vi "PPG_ABC.set letter time.vi"(0 "i ref in":refnum<vi>, 1 "letter":string, 2 "time [us]":dbl, 3 "ms timeout [ms]":i32=10000, 4 "patternGroup":i32, 5 "error in (no error)":errorcluster) -> (14 "i ref out":refnum<vi>, 17 "timed out":bool, 19 "error out":errorcluster)   [LabVIEW 2014, in "PPG_ABC.lvlib"]
doc: "Recalculates and reloads actual patterns for given letter and time. This routine can only by used, after patterns have been loaded using the method \"LoadABC\"."
uses:
  PPG_ABC.lvlib
  CS_Core/CSSystem/CoreDefs/CoreDefs.error_type.ctl
  CS_Core/CSSystem/CoreDefs/CoreDefs.error_severity.ctl
  CS_Core/CSSystem/CoreLib/CoreLib.lvlib
  CSlibraries/UtilityLib/UtilityLib.lvlib
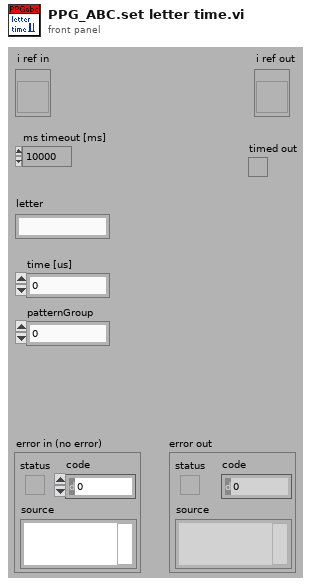
[diagram p1: front panel]
types:
  T1 = typedef "CoreDefs.error_severity.ctl" = enum16{"undefined", "information", "warning", "error", "fatal"}
  T2 = typedef "CoreDefs.error_type.ctl" = enum16{"no error", "can't load process", "can't unload process", "process does not exist", "can't install process", "can't remove process", "unknown function", "time out", "can't execute function", "duplicate queue name", "super not found", "caller queue invalid", "can't ping process", "unknown error", "VISA Error", "VISA timeout", "GPIB timeout", "GPIB error", "communication error", "data type mismatch", "can't read data from OPC server", "can't write data to OPC server", "OET error", "function not implemented", "process already exists", "invalid Shared Variable name", "error writing Shared Variable", "error reading Shared Variable", "invalid client name", "corrupt database", "unknown class", "call not authorized", "parameter out of range", "OET timeout: can't get data to modify", "invalid queue name", "requested operation incompatible with current state", "event undefined", "event disabled", "state undefined", "caller is not a friend", "EventBuilder: bad eventID", "EventBuilder: no DAQ devices", "a thread must not stop itself", "UNUSED ELEMENT4", "DiscArchiver: eventData incomplete", "DiscArchiver: eventData does not belong to run", "DiscArchiver: can't open file", "DiscArchiver: can't write to file", "DiscArchiver: available disc space low", "can't acquire semaphore", "error reading data from database", "notifier object is not existing", "can't register process", "can't unregister process", "illegal event type", "object disabled", "object already exists", "can't change state", "Instrument not found", "no connection to remote node", "invalid reference", "N/A", "UNUSED ELEMENT 1", "element not found", "illegal TCP/IP connection detected", "object does not exist", "invalid access ID", "unknown CS system", "invalid privilige", "unsupported data type", "unsupported server type", "IO server already exists", "Shared Variable already exists"}
  T3 = typedef "PPG_ABC.lvlib/PPG_ABC.i attribute.ctl" = cluster{"patternGroups":T4[], "defaultLetter":string, "defaultPatternGroup":i32, "PGRunning":T5, "PGRunningID":i32, "pgStarting":T6}
  T4 = typedef "PPG_ABC.lvlib/PPG_ABC.PG_dataType.ctl" = cluster{"PGDevice":string, "rawPatternData":cluster{"triggerCondition":i32, "timeTable":dbl[], "channelTable":string[]}[]}
  T5 = typedef "PPG_ABC.lvlib/PPG_ABC.PG_Running.ctl" = i32
  T6 = typedef "Semaphore RefNum" = refnum<k1>
  T7 = cluster{"triggerCondition":i32, "timeTable":dbl[], "channelTable":string[]}[]
  T8 = cluster{"triggerCondition":i32, "timeTable":dbl[], "channelTable":string[]}
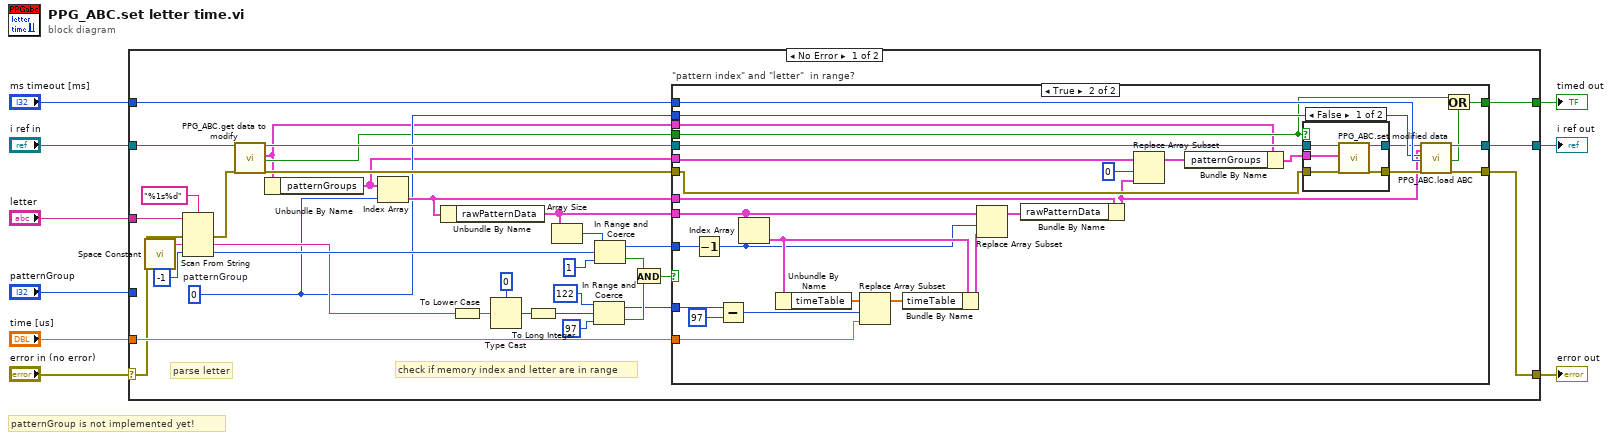
[diagram p0: block diagram]
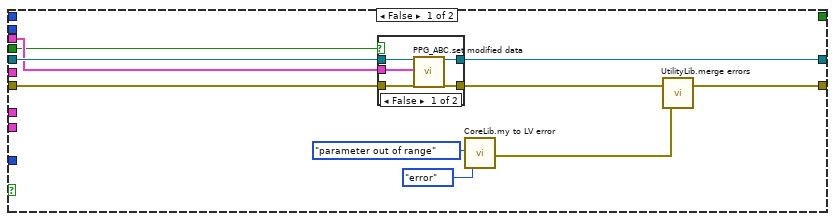
[diagram p2: hidden frame]
diagram:
  # "patternGroup is not implemented yet!"
  n1 = case shown="No Error" "error in (no error)" {
    selector: "error in (no error)" -> [w13 w100]
    tunnel: [w22 w100] -> w8
    tunnel: "i ref in" -> [w40 w99]
    tunnel: [w24 w99] -> w6
    tunnel: "ms timeout [ms]" -> [w20 _]
    tunnel: "letter" -> [w44 _]
    tunnel: "time [us]" -> [w21 _]
    tunnel: [w19 _] -> w2
    tunnel: "patternGroup" -> [_ _]
    frame No Error {
      w14 = 0  # patternGroup
      # "check if memory index and letter are in range"
      # "parse letter"
      n2 = call <vilib>:"Space Constant.vi"() -> ("String"=w42:string)
      n3 = Scan From String(format string="%1s%d", input string=w44, error in=w13, default 1=w42, default 2=-1 ("default value 2")) -> (error out=w38:errorcluster, output 1=w33:string, output 2=w35:i32)  [unwired: 1 in, 2 out]
      n4 = call "PPG_ABC.get data to modify.vi"("i ref in"=w40, "error in (no error)"=w38) -> ("i ref out"=w39:refnum<vi>, "i attribute"=w10:T3, "timed out"=w12:bool, "error out"=w23:errorcluster)  [unwired: 14 in]
      n5 = Unbundle By Name(w10) -> ("patternGroups"=w11:T4[])
      n6 = Index Array(array=w11, index=w14) -> (element=w15:T4)
      n7 = Unbundle By Name(w15) -> ("rawPatternData"=w16:T7)
      n8 = To Lower Case(string=w33) -> (all lower case string=w18:string)
      n9 = Type Cast(type=u8 0, x=w18) -> (*(type *) &x=w32:u8)
      n10 = To Long Integer(number=w32) -> (32bit integer=w17:i32)
      n11 = Array Size(array=w16) -> (size(s)=w37:i32)
      n12 = In Range and Coerce(upper limit=122, x=w17, lower limit=97) -> (coerced(x)=w25:i32, In Range?=w26:bool)
      n13 = In Range and Coerce(upper limit=w37, x=w35, lower limit=1) -> (coerced(x)=w34:i32, In Range?=w27:bool)
      n14 = And(x=w27, y=w26) -> (x .and. y?=w28:bool)
      n15 = case "\"pattern index\" and \"letter\"  in range?" shown="True" w28 {
        tunnel: w39 -> [w48 w73]
        tunnel: w34 -> [_ w91]
        tunnel: w25 -> [_ w90]
        tunnel: [w47 w83] -> w24
        tunnel: w23 -> [w50 w68]
        tunnel: [w52 w82] -> w22
        tunnel: w21 -> [_ w89]
        tunnel: w20 -> [_ w81]
        tunnel: [_ w71] -> w19
        tunnel: w16 -> [_ w77]
        tunnel: w15 -> [_ w76]
        tunnel: w14 -> [_ w75]
        tunnel: w12 -> [w45 w69]
        tunnel: w11 -> [_ w67]
        tunnel: w10 -> [w46 w64]
        frame False {
          n16 = case shown="False" w45 {
            tunnel: w50 -> [w59 w60]
            tunnel: [w58 w60] -> w49
            tunnel: w48 -> [w57 w61]
            tunnel: [w56 w61] -> w47
            tunnel: w46 -> [w55 _]
            frame False {
              n17 = call "PPG_ABC.set modified data.vi"("i ref in"=w57, "i attribute"=w55, "error in (no error)"=w59) -> ("i ref out"=w56:refnum<vi>, "error out"=w58:errorcluster)  [unwired: 15 in]
            }
            frame True {
            }
          }
          n18 = call "CoreLib.my to LV error.vi"("ErrorTypes"=CoreDefs.error_type."parameter out of range", "severityLevel"=CoreDefs.error_severity."error") -> ("myErrorCluster"=w51:errorcluster)  [unwired: 16 in, 1 out]
          n19 = call "UtilityLib.merge errors.vi"("error2 (no error)"=w51, "error1 (no error)"=w49) -> ("error out"=w52:errorcluster)
        }
        frame True {
          n20 = Decrement(x=w91) -> (x-1=w78:i32)
          n21 = Subtract(x=w90, y=97) -> (x-y=w80:i32)
          n22 = Index Array(array=w77, index=w78) -> (element=w87:T8)
          n23 = Unbundle By Name(w87) -> ("timeTable"=w88:dbl[])
          n24 = Replace Array Subset(array=w88, new element=w89, index=w80) -> (w86:dbl[])
          n25 = Bundle By Name(cluster=w87, "timeTable"=w86) -> (w85:T8)
          n26 = Replace Array Subset(array=w77, new element=w85, index=w78) -> (w84:T7)
          n27 = Bundle By Name(cluster=w76, "rawPatternData"=w84) -> (w66:T4)
          n28 = Replace Array Subset(array=w67, new element=w66, index=0) -> (w63:T4[])
          n29 = Bundle By Name(cluster=w64, "patternGroups"=w63) -> (w62:T3)
          n30 = case shown="False" w69 {
            tunnel: w68 -> [w96 w97]
            tunnel: [w95 w97] -> w74
            tunnel: w73 -> [w94 w98]
            tunnel: [w93 w98] -> w72
            tunnel: w62 -> [w92 _]
            frame False {
              n31 = call "PPG_ABC.set modified data.vi"("i ref in"=w94, "i attribute"=w92, "error in (no error)"=w96) -> ("i ref out"=w93:refnum<vi>, "error out"=w95:errorcluster)  [unwired: 15 in]
            }
            frame True {
            }
          }
          n32 = call "PPG_ABC.load ABC.vi"("i ref in"=w72, "PGData"=w66, "patternGroup"=w75, "ms timeout [ms]"=w81, "error in (no error)"=w74) -> ("i ref out"=w83:refnum<vi>, "timed out"=w70:bool, "error out"=w82:errorcluster)  [unwired: 12 in]
          n33 = Or(x=w69, y=w70) -> (x .or. y?=w71:bool)
        }
      }
    }
    frame Error {
    }
  }
  "error out" <- w8
  "i ref out" <- w6
  "timed out" <- w2
